vi "Update Node State.vi"(7 "Received Tick":u32, 8 "error in":errorcluster, 9 "Frame Data":u8[](array[numeric]) format="%02x", 10 "Node ID":u8, 11 "Node Guard in":refnum<class "Node Guard.lvclass">) -> (0 "error out":errorcluster, 3 "Node Guard out":refnum<class "Node Guard.lvclass">)   [LabVIEW 2020, in "CANopen.lvlib" / "Network Management.lvlib" / "Node Guard.lvlib" / "Node Guard.lvclass"]
uses:
  Node Guard.lvclass
  Node Guard.lvclass/Node Guard.ctl
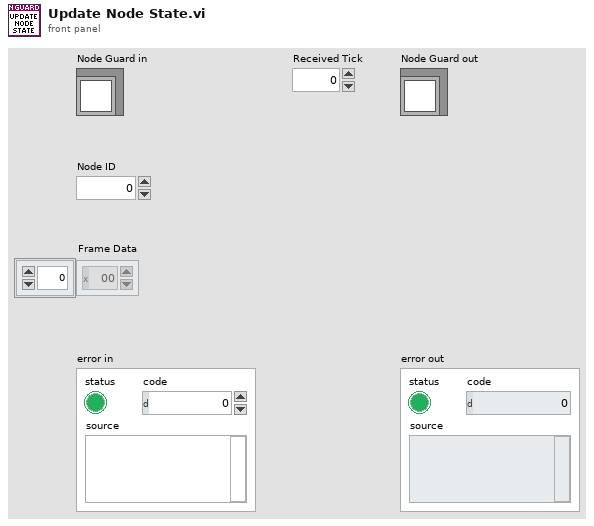
[diagram p1: front panel]
types:
  T1 = map{u8, cluster{"State":u8, "Timings":cluster{"Guard time (ms)":u32, "Lifetime Factor":dbl}, "Toogle Bit":bool, "Delivery Notifier":refnum<notifier>, "Last Received Tick":u32}}
  T2 = cluster{"State":u8, "Timings":cluster{"Guard time (ms)":u32, "Lifetime Factor":dbl}, "Toogle Bit":bool, "Delivery Notifier":refnum<notifier>, "Last Received Tick":u32}
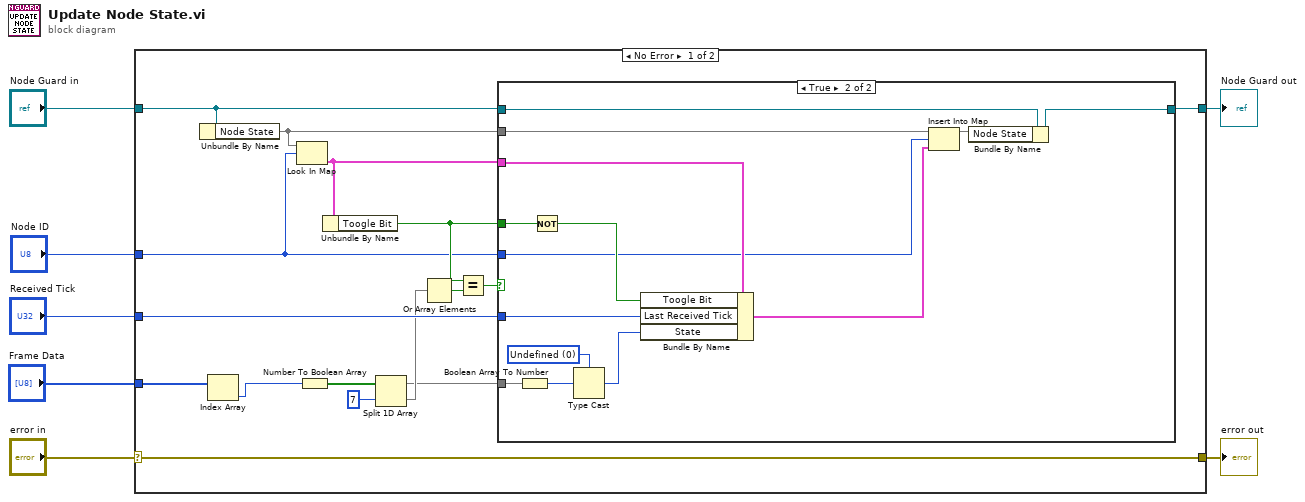
[diagram p0: block diagram]
diagram:
  n1 = case shown="No Error" "error in" {
    selector: "error in" -> [w23 w40]
    tunnel: [w23 w40] -> w4
    tunnel: [w21 w39] -> w6
    tunnel: "Node Guard in" -> [w22 w39]
    tunnel: "Node ID" -> [w9 _]
    tunnel: "Frame Data" -> [w18 _]
    tunnel: "Received Tick" -> [w20 _]
    frame No Error {
      n2 = Unbundle By Name(w22) -> ("Node State"=w8:T1)
      n3 = Index Array(array=w18) -> (element=w14:u8)  [unwired: 1 in]
      n4 = Look In Map(map=w8, key=w9) -> (value=w19:T2)  [unwired: 1 in, 1 out]
      n5 = Number To Boolean Array(number=w14) -> (Boolean array=w17:bool[])
      n6 = Unbundle By Name(w19) -> ("Toogle Bit"=w10:bool)
      n7 = Split 1D Array(array=w17, index=7) -> (first subarray=w13:bool[], second subarray=w15:bool[])
      n8 = Or Array Elements(Boolean array=w15) -> (logical OR=w11:bool)
      n9 = Equal?(x=w10, y=w11) -> (x = y?=w12:bool)
      n10 = case shown="True" w12 {
        tunnel: w22 -> [w24 w38]
        tunnel: [w24 w37] -> w21
        tunnel: w20 -> [_ w35]
        tunnel: w19 -> [_ w30]
        tunnel: w13 -> [_ w34]
        tunnel: w10 -> [_ w29]
        tunnel: w9 -> [_ w26]
        tunnel: w8 -> [_ w25]
        frame False {
        }
        frame True {
          w31 = u8 0 items=["Undefined"=0, "Stopped"=4, "Operational"=5, "Pre-operational"=127] ("State")
          n11 = Boolean Array To Number(Boolean array=w34) -> (number=w33:u32)
          n12 = Not(x=w29) -> (.not. x?=w28:bool)
          n13 = Type Cast(type=w31, x=w33) -> (*(type *) &x=w32:u8)
          n14 = Bundle By Name(cluster=w30, "Toogle Bit"=w28, "Last Received Tick"=w35, "State"=w32) -> (w27:T2)
          n15 = Insert Into Map(map in=w25, key=w26, value=w27) -> (map out=w36:T1)  [unwired: 2 out]
          n16 = Bundle By Name(cluster=w38, "Node State"=w36) -> (w37:refnum<class "Node Guard.lvclass">)
        }
      }
    }
    frame Error {
    }
  }
  "Node Guard out" <- w6
  "error out" <- w4
